vi "example_01_xml_convert.vi"() -> ()   [LabVIEW 2015, in "lv-unit-conversion.lvlib"]
uses:
  lv-unit-conversion.lvlib
  public/advanced/load_dictionary_xml.vi
panel:
  out "time_to_read":dbl format="%<%H:%M:%S%3u>t"
  out "value out":dbl
  in  "value in":dbl
  in  "source_unit":string="m"
  in  "conversion_unit":string="in"
  out "unit_dictionary":variant
  out "error out":errorcluster
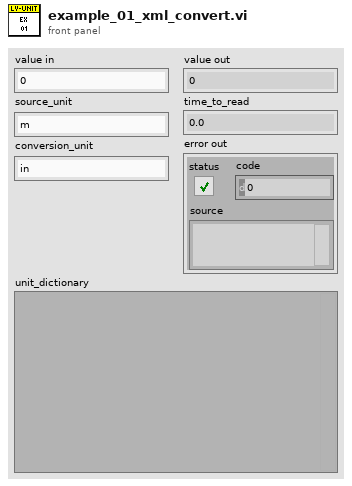
[diagram p1: front panel]
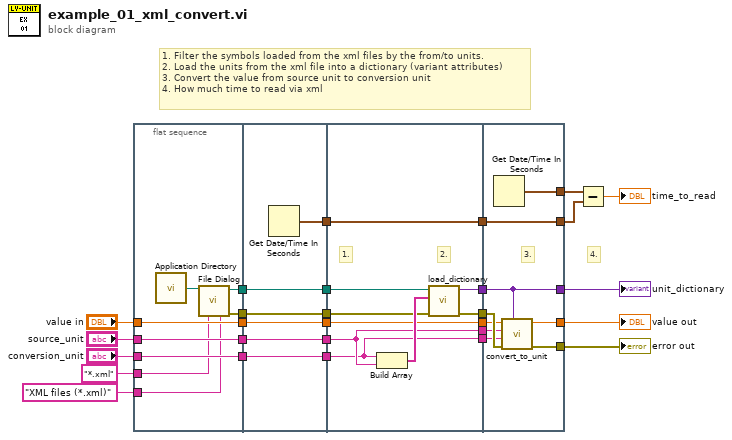
[diagram p0: block diagram]
diagram:
  # "4."
  # "1. Filter the symbols loaded from the xml files by the from/to units.\n2. Load the units from the xml file into a dictionary (variant attributes)\n3. Convert the value from source unit to conversion unit\n4. How much time to read via xml"
  n1 = flat-sequence {
    tunnel: "value in" -> [w34]
    tunnel: "conversion_unit" -> [w35]
    tunnel: "source_unit" -> [w36]
    tunnel: [w36] -> w11
    tunnel: [w35] -> w9
    tunnel: [w34] -> w7
    tunnel: [w33] -> w4
    tunnel: [w32] -> w2
    tunnel: "*.xml" ("pattern (all files)") -> [w31]
    tunnel: "XML files (*.xml)" ("pattern label") -> [w30]
    tunnel: w11 -> [w42]
    tunnel: [w42] -> w10
    tunnel: w9 -> [w41]
    tunnel: [w41] -> w8
    tunnel: w7 -> [w40]
    tunnel: [w40] -> w6
    tunnel: [w37] -> w5
    tunnel: w4 -> [w39]
    tunnel: [w39] -> w3
    tunnel: w2 -> [w38]
    tunnel: [w38] -> w1
    tunnel: [w51] -> w24
    tunnel: [w50] -> w23
    tunnel: [w48] -> w22
    tunnel: [w47] -> w21
    tunnel: [w46] -> w20
    tunnel: [w45] -> w17
    tunnel: w10 -> [w47]
    tunnel: w8 -> [w46]
    tunnel: w6 -> [w48]
    tunnel: w5 -> [w45]
    tunnel: w3 -> [w44]
    tunnel: w1 -> [w43]
    tunnel: [w59] -> w26
    tunnel: w24 -> [w60]
    tunnel: w23 -> [w59]
    tunnel: w22 -> [w58]
    tunnel: w21 -> [w57]
    tunnel: w20 -> [w56]
    tunnel: [w55] -> w19
    tunnel: [w54] -> w18
    tunnel: w17 -> [w53]
    tunnel: [w53] -> w15
    tunnel: [w52] -> w16
    frame #0 {
      n2 = call <vilib>:"Application Directory.vi"() -> ("Application Directory"=w29:path)
      n3 = call "File Dialog"("start path"=w29, "pattern (all files)"=w31, "pattern label"=w30) -> ("selected path"=w32:path, "error out"=w33:errorcluster)  [unwired: 9 in, 2 out]
    }
    frame #1 {
      n4 = Get Date/Time In Seconds() -> (seconds since 1Jan1904=w37:timestamp)
    }
    frame #2 {
      # "2."
      # "1."
      n5 = Build Array(w46, w47) -> (w49:string[])
      n6 = call-poly "load_dictionary.vi"("error in (no error)"=w44, "symbols []"=w49, "xml_path"=w43) -> ("error out"=w51:errorcluster, "unit_dictionary"=w50:variant)  [unwired: 7 in]
    }
    frame #3 {
      # "3."
      n7 = Get Date/Time In Seconds() -> (seconds since 1Jan1904=w52:timestamp)
      n8 = call "convert_to_unit.vi"("unit_dictionary"=w59, "error in (no error)"=w60, "unit_to"=w56, "unit_from"=w57, "value in"=w58) -> ("error out"=w54:errorcluster, "value out"=w55:dbl)  [unwired: 5 in]
    }
  }
  n9 = Subtract(x=w16, y=w15) -> (x-y=→"time_to_read":dbl)
  "error out" <- w18
  "unit_dictionary" <- w26
  "value out" <- w19
